vi "synchronize.vi"(8 "error in (no error)":errorcluster, 10 "Received frame In":cdb[][](array[numeric])=array1x226352[226352 elements], 11 "Synchronizer in":refnum<class "Synchronizer.lvclass">) -> (0 "error out":errorcluster, 1 "Detected?":bool=TRUE, 2 "Received frame Out":cdb[][](array[numeric]), 3 "Synchronizer out":refnum<class "Synchronizer.lvclass">, 4 "NextOffset":i32, 5 "Peak Position":i32=513)   [LabVIEW 2012, in "Synchronizer.lvclass"]
uses:
  Synchronizer.lvclass
  Synchronizer.lvclass/Synchronizer.ctl
  <vilib>/Analysis/5stat.llb/RMS (CDB).vi
  <vilib>/Analysis/2dsp.llb/1D Convolution (CDB).vi
  <vilib>/Analysis/2dsp.llb/Decimate (single shot, CDB).vi
  <vilib>/Analysis/NI_AALPro.lvlib
panel:
  out "Synchronization magnitude":dbl[](graph)
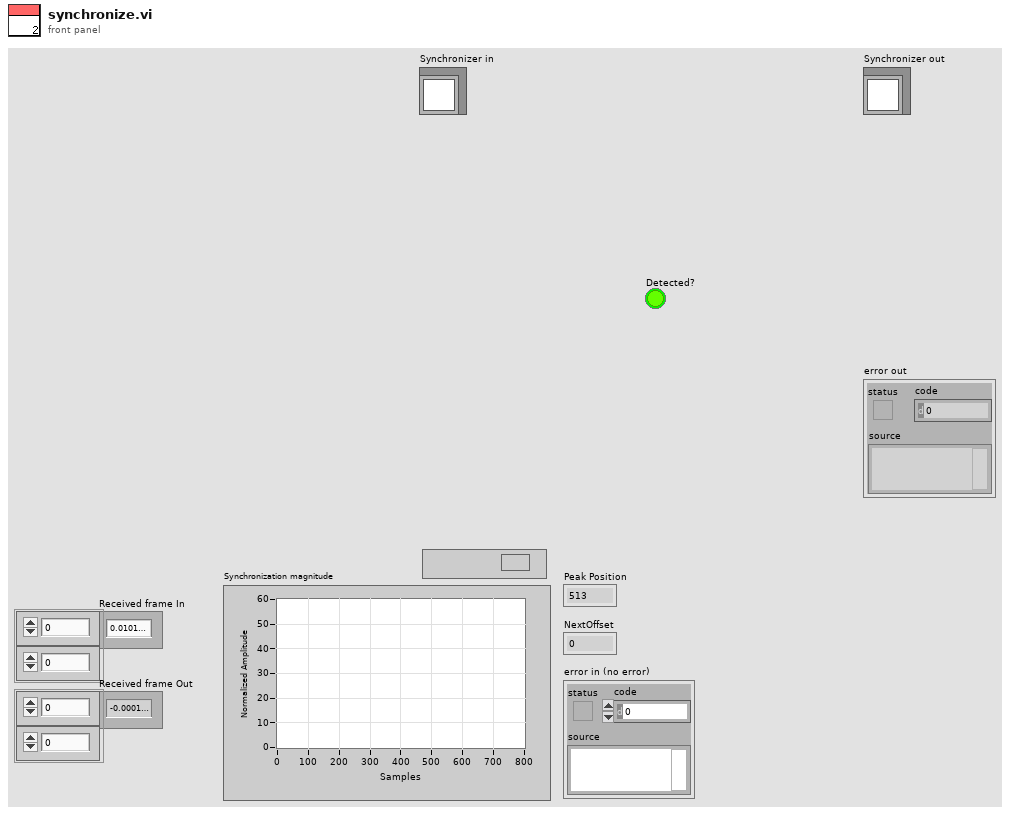
[diagram p1: front panel]
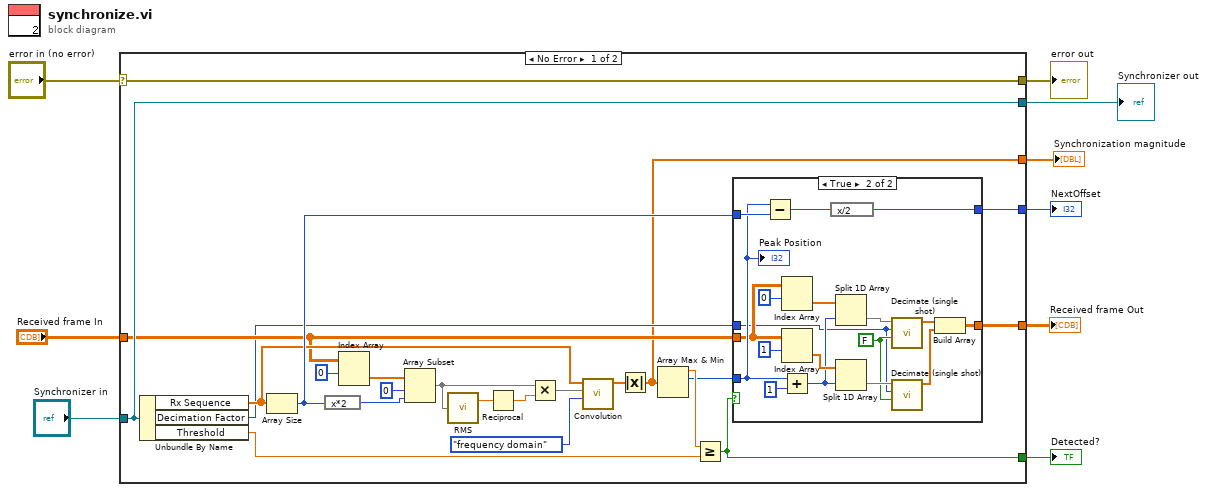
[diagram p0: block diagram]
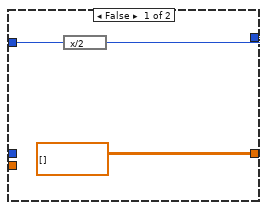
[diagram p2: hidden frame]
diagram:
  n1 = case shown="No Error" "error in (no error)" {
    selector: "error in (no error)" -> [w32 w55]
    tunnel: [w32 w55] -> w8
    tunnel: [w18 w54] -> w6
    tunnel: "Synchronizer in" -> [w18 w54]
    tunnel: "Received frame In" -> [w16 _]
    tunnel: [w13 _] -> w4
    tunnel: [w12 _] -> w3
    tunnel: [w11 _] -> w2
    tunnel: [w10 _] -> w1
    frame No Error {
      n2 = Unbundle By Name(w18) -> ("Rx Sequence"=w17:cdb[], "Decimation Factor"=w15:u8, "Threshold"=w14:dbl)
      n3 = Array Size(array=w17) -> (size(s)=w25:i32)
      n4 = expression code="x*2"(w25) -> (w28:i32)
      n5 = Index Array(array=w16, index (row)=0) -> (element=w21:cdb[])  [unwired: 1 in]
      n6 = Array Subset(array=w21, index=0, length=w28) -> (w23:cdb[])
      n7 = call-poly <vilib>:"RMS.vi"("X"=w23) -> ("rms value"=w27:dbl)  [unwired: 1 out]
      n8 = Reciprocal(x=w27) -> (1/x=w19:dbl)
      n9 = Multiply(x=w23, y=w19) -> (x*y=w24:cdb[])
      n10 = call-poly <vilib>:"Convolution.vi"("algorithm"=enum32{"direct", "frequency domain"}."frequency domain", "Y"=w24, "X"=w17) -> ("X * Y"=w20:cdb[])  [unwired: 7 in, 1 out]
      n11 = Absolute Value(x=w20) -> (abs(x)=w13:dbl[])
      n12 = Array Max & Min(array=w13) -> (max value=w30:dbl, max index (indices)=w29:i32)  [unwired: 2 out]
      n13 = Greater Or Equal?(x=w30, y=w14) -> (x >= y?=w10:bool)
      n14 = case shown="True" w10 {
        tunnel: w29 -> [_ w52]
        tunnel: w25 -> [w33 w53]
        tunnel: w16 -> [_ w46]
        tunnel: [cdb[][] [] w42] -> w11
        tunnel: [w34 w51] -> w12
        tunnel: w15 -> [_ w36]
        frame False {
          n15 = expression code="x/2"(w33) -> (w34:i32)
        }
        frame True {
          w38 = FALSE ("averaging")
          n16 = Subtract(x=w52, y=w53) -> (x-y=w50:i32)
          n17 = Index Array(array=w46, index (row)=0) -> (element=w45:cdb[])  [unwired: 1 in]
          n18 = Index Array(array=w46, index (row)=1) -> (element=w44:cdb[])  [unwired: 1 in]
          n19 = Add(x=w52, y=1) -> (x+y=w43:i32)
          n20 = expression code="x/2"(w50) -> (w51:i32)
          n21 = Split 1D Array(array=w45, index=w43) -> (second subarray=w41:cdb[])  [unwired: 1 out]
          n22 = Split 1D Array(array=w44, index=w43) -> (second subarray=w39:cdb[])  [unwired: 1 out]
          n23 = call-poly <vilib>:"Decimate (single shot).vi"("averaging"=w38, "decimating factor"=w36, "X"=w41) -> ("Decimated Array"=w40:cdb[])  [unwired: 7 in, 1 out]
          n24 = call-poly <vilib>:"Decimate (single shot).vi"("averaging"=w38, "decimating factor"=w36, "X"=w39) -> ("Decimated Array"=w37:cdb[])  [unwired: 7 in, 1 out]
          n25 = Build Array(w40, w37) -> (w42:cdb[][])
          "Peak Position" <- w52
        }
      }
    }
    frame Error {
    }
  }
  "error out" <- w8
  "Synchronizer out" <- w6
  "Synchronization magnitude" <- w4
  "NextOffset" <- w3
  "Received frame Out" <- w2
  "Detected?" <- w1
